vi "RT Main_EVO_V1_chopped_data_V1.vi"(11 "dup Message Queue 2":refnum<queue>) -> ()   [LabVIEW 2017]
uses:
  UI Error Handlers/support/Message Queue/Message Cluster.ctl
  <vilib>/vision/Image Controls.llb/IMAQ Image.ctl
  <vilib>/userdefined/High Color/IMAQdx.ctl
  <vilib>/vision/Avi.llb/IMAQ AVI2 Refnum.ctl
  camera_array_1.ctl
  <vilib>/vision/Avi.llb/IMAQ AVI2 Codec Path.ctl
  Globals/Global - All RT Loop Stop.vi
  Globals/Global - Configuration Options.vi
  <vilib>/vision/driver/NI_Vision_Acquisition_Software.lvlib
  UI Error Handlers/support/Message Queue/Message Queue.lvlib
panel:
  in  "Boolean":bool
  out "Array":T1[](array[typedef])
  out "Webcam":T1(plugin-control)
  out "Codec Names 2":string[](array[string])
  out "concatenated string 4":string
  out "error out":errorcluster
  out "x-y":u32
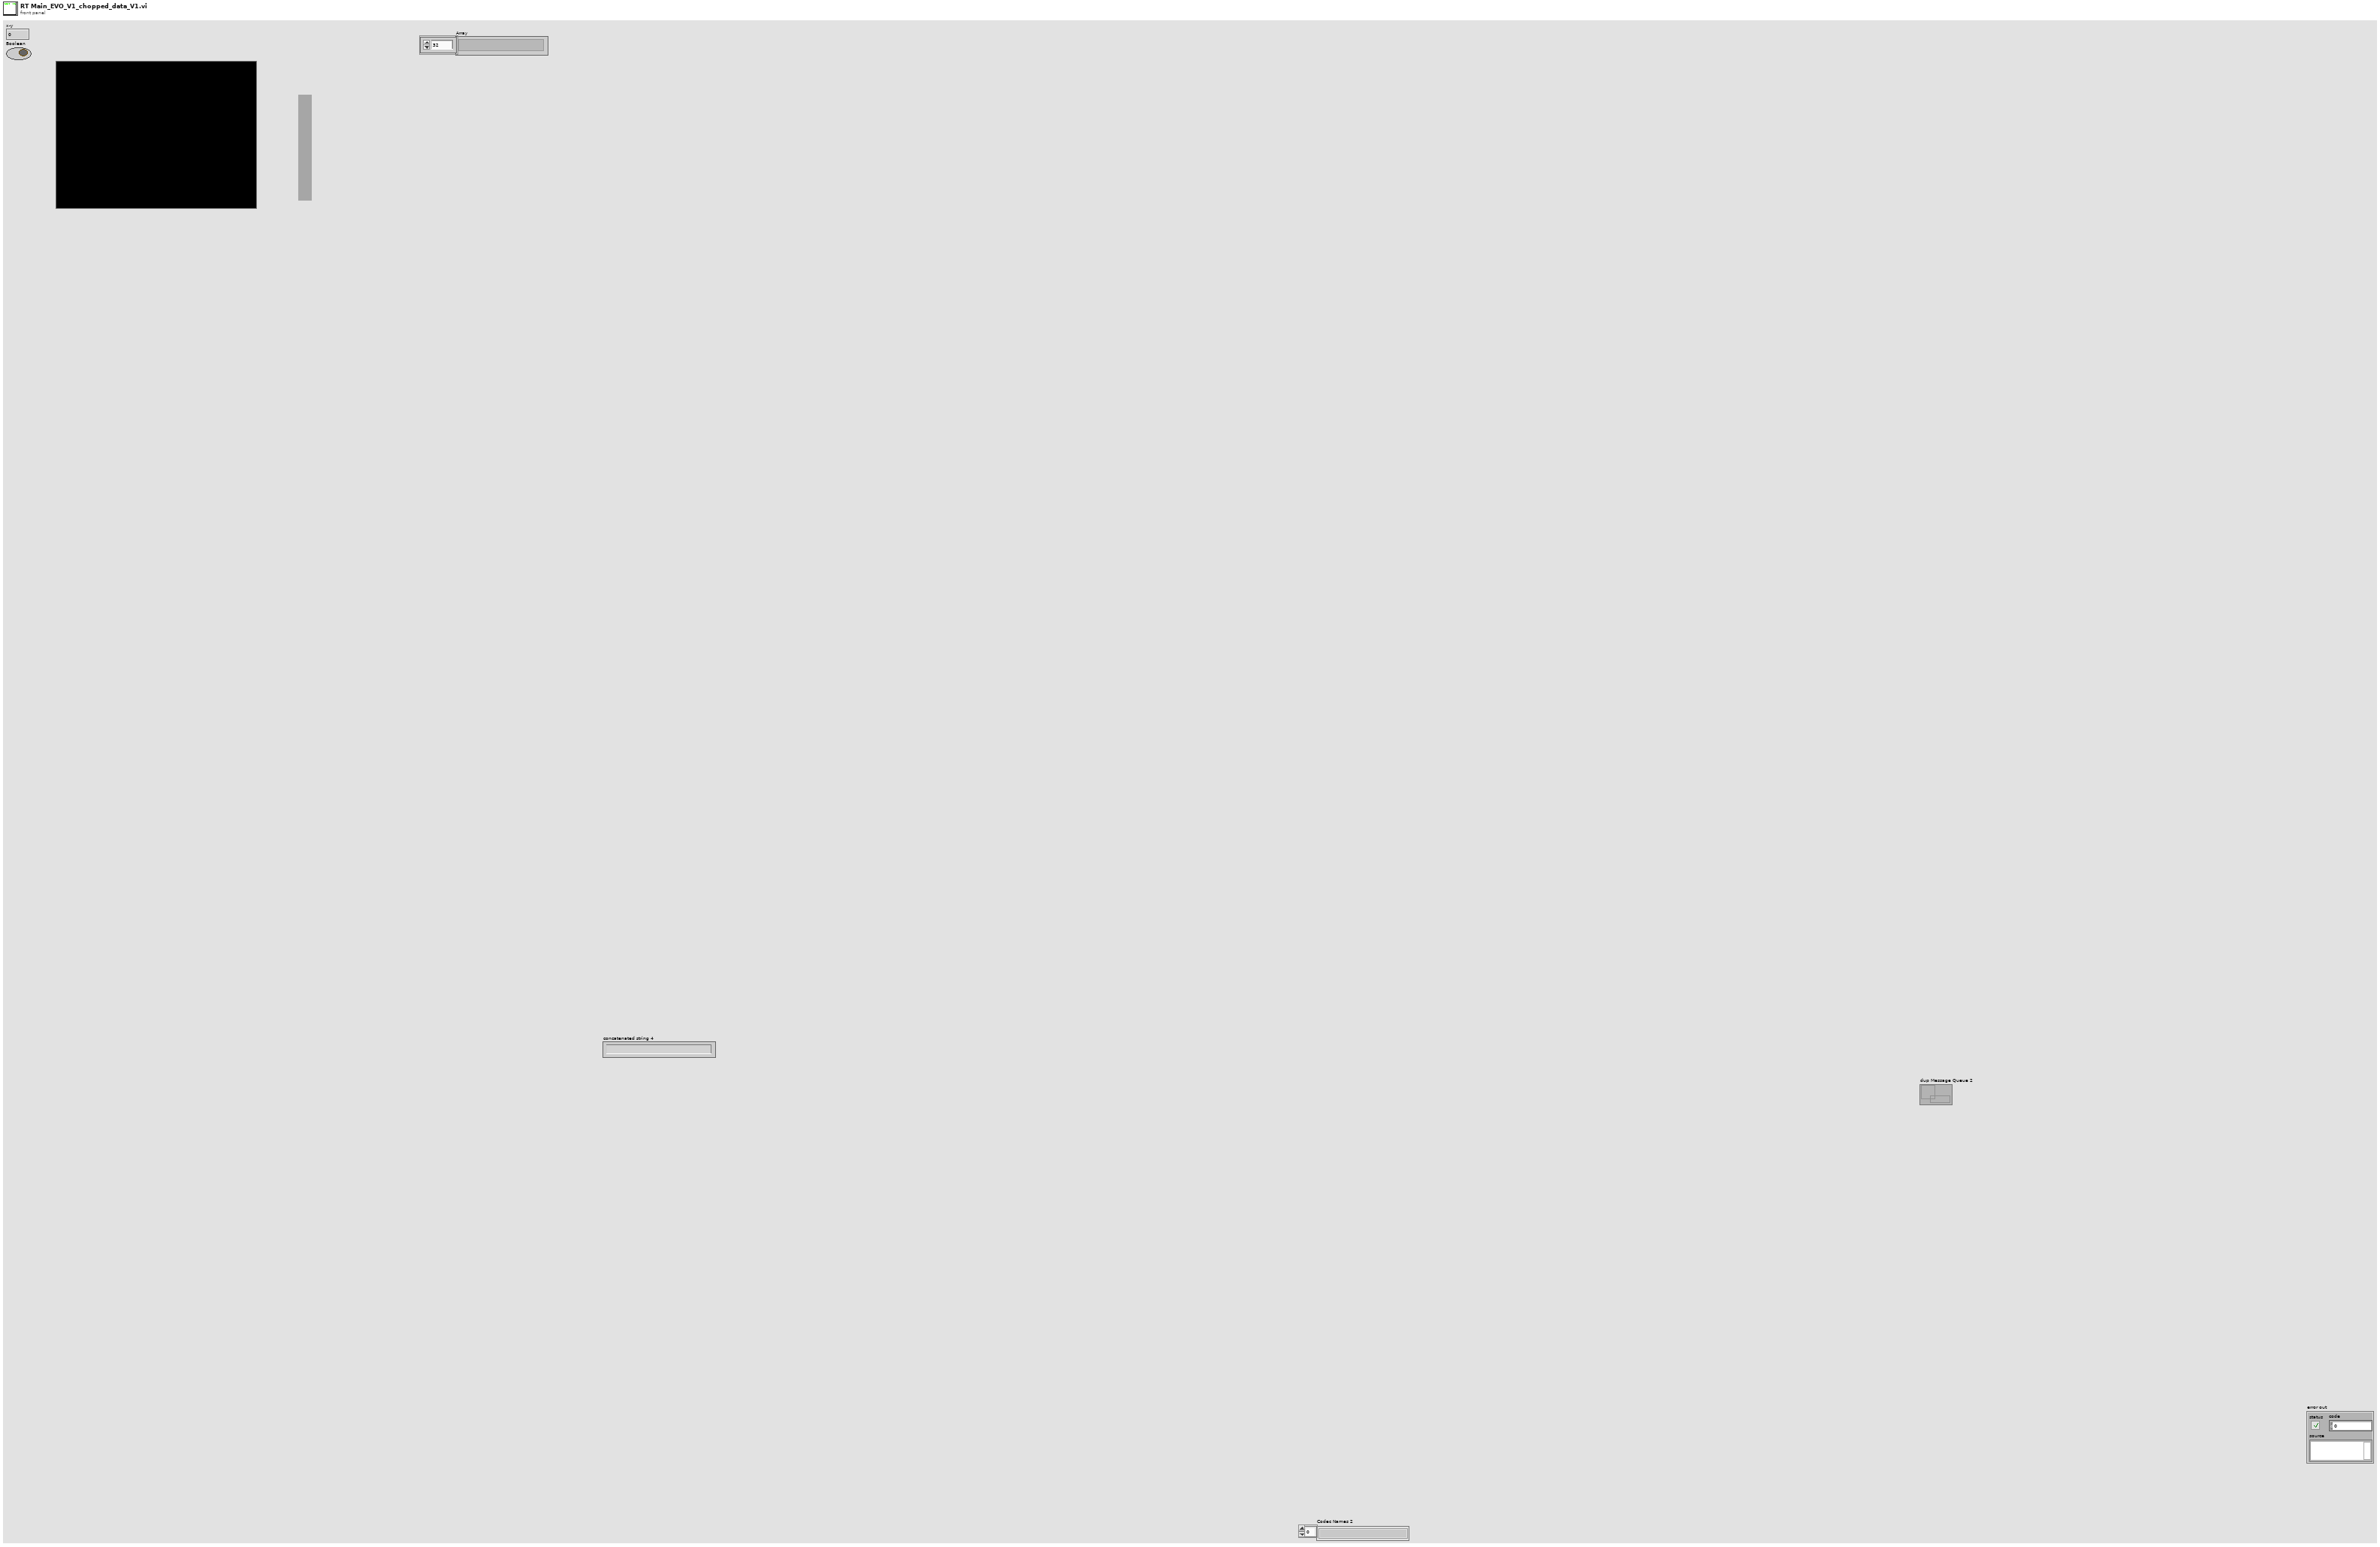
[diagram p1: front panel]
types:
  T1 = typedef "IMAQ Image.ctl" = refnum<image>
  T2 = typedef "camera_array_1.ctl" = T1[]
  T3 = typedef "IMAQ AVI2 Refnum.ctl" = refnum<k20>
  T4 = typedef "IMAQdx.ctl" = refnum<k21>
  T5 = typedef "Image Type" = u32
  T6 = cluster{"Tool data":cluster{"Number of teeth":sgl}, "Cutting data":cluster{"rpm":sgl}, "Limits":cluster{"Magnitude threshold":sgl, "Tolerance":sgl}, "G1 status":cluster{"G1 trigger":bool}}
  T7 = typedef "IMAQ AVI2 Codec Path.ctl" = u32
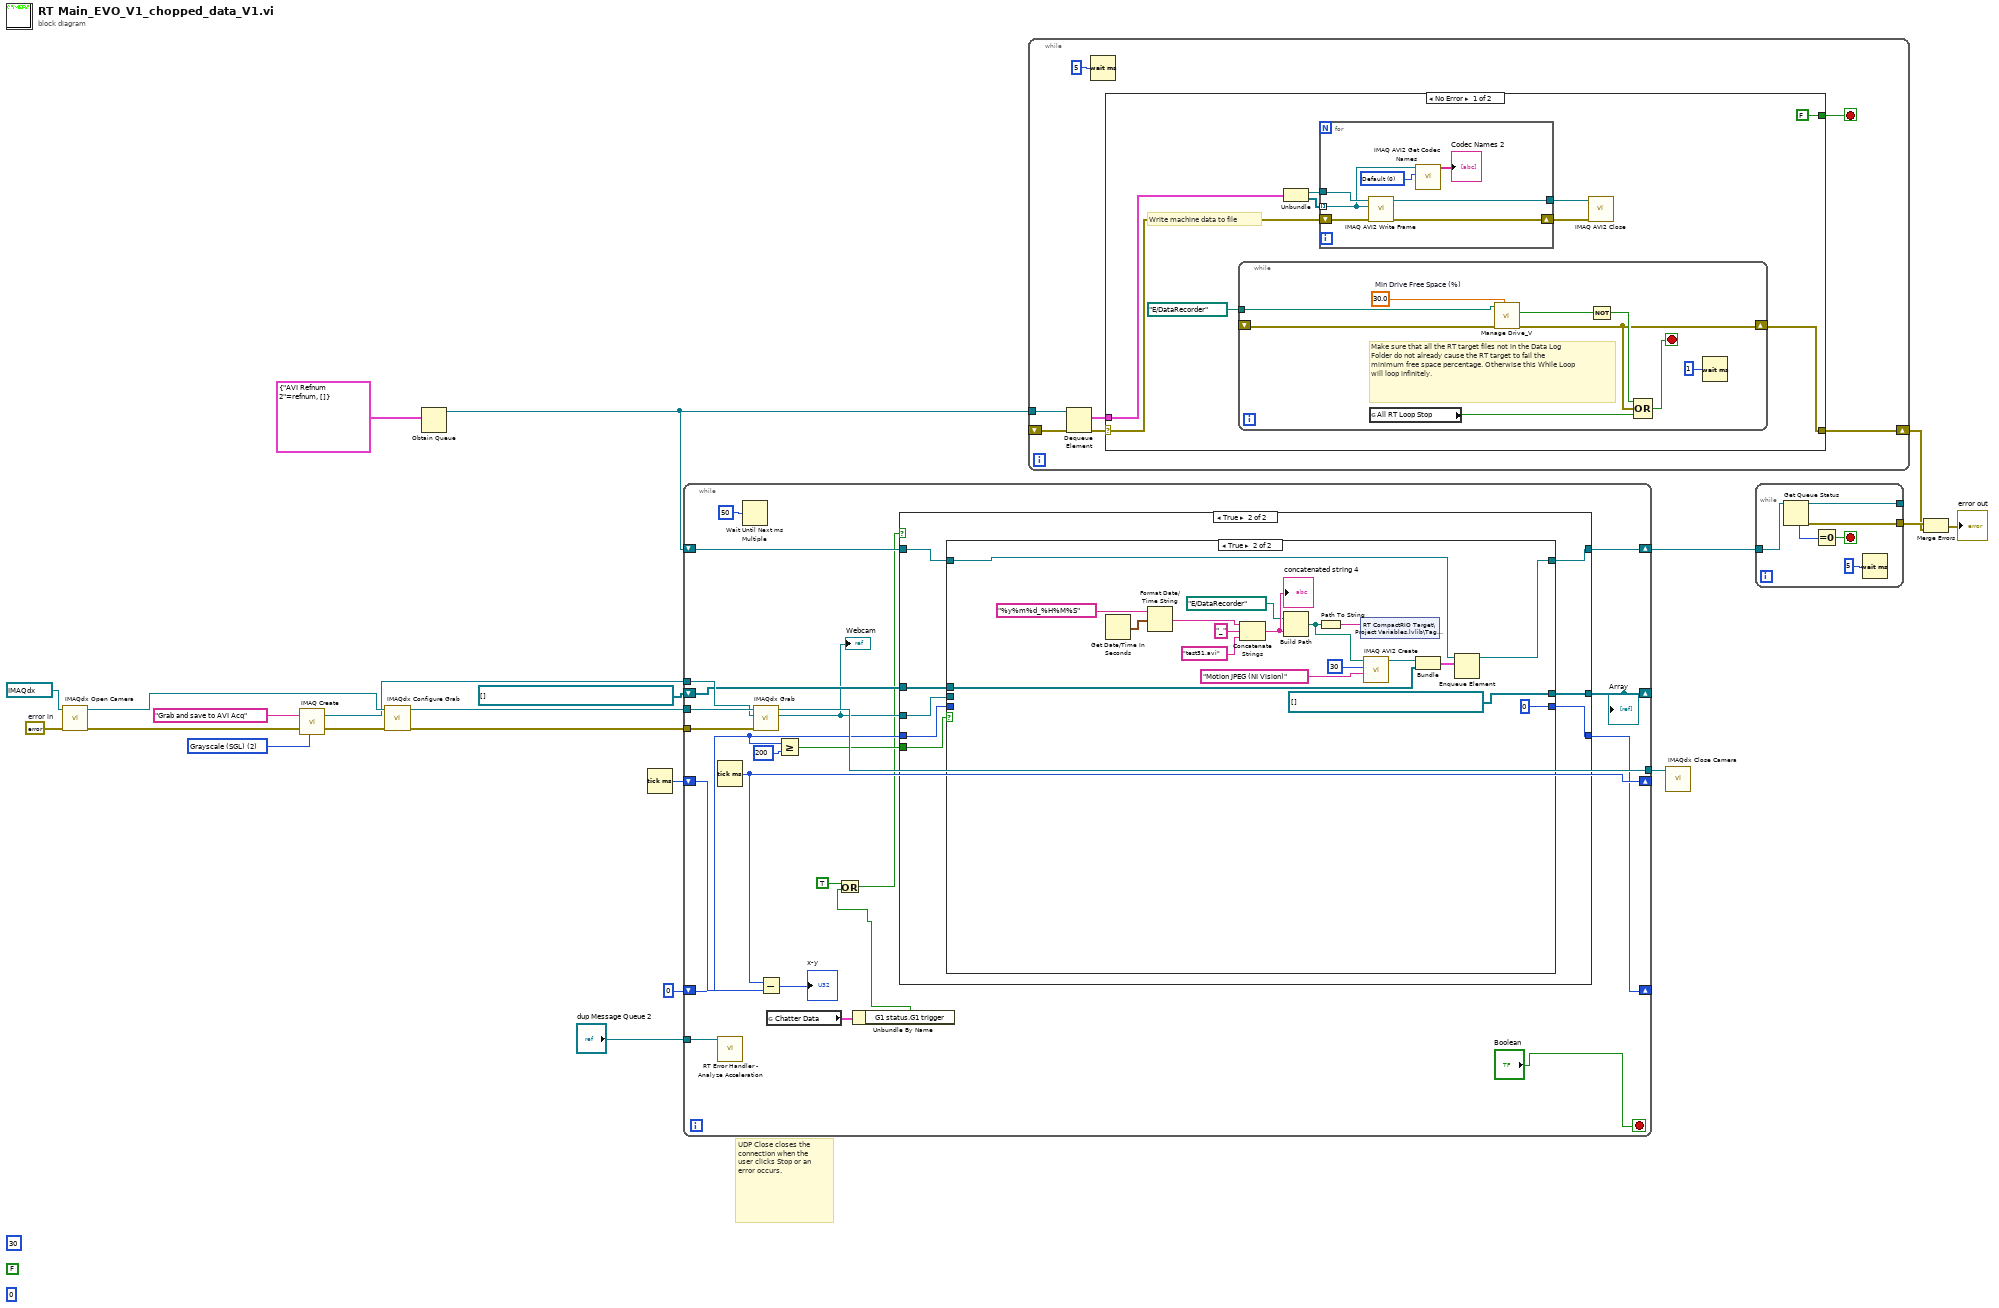
[diagram p0: block diagram]
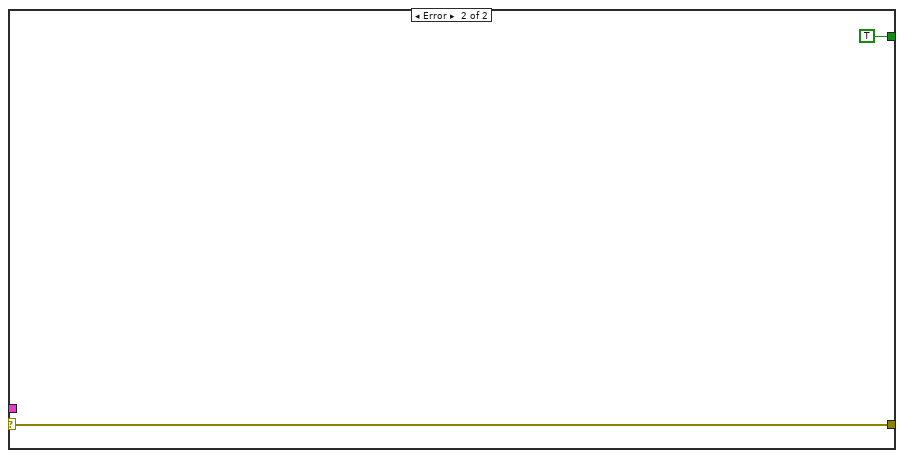
[diagram p2: hidden frame]
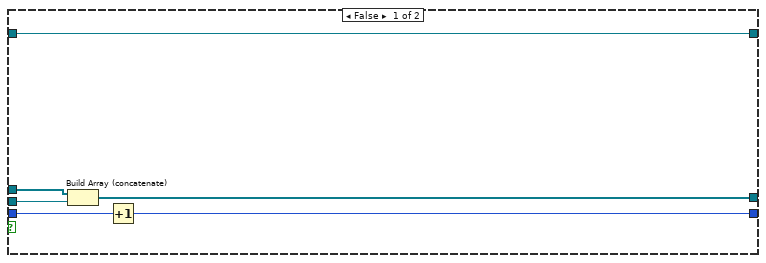
[diagram p4: hidden frame]
diagram:
  w11 = T5 2 items=["Grayscale (U8)", "Grayscale (I16)", "Grayscale (SGL)", "Complex (CSG)", "RGB (U32)", "HSL (U32)", "RGB (U64)", "Grayscale (U16)"] ("Image Type")
  (unwired) u32 30 ("Frames Per Second")
  w12 = errorcluster {"status"=FALSE, "code"=0, "source"=""}  # error in
  (unwired) i16 0 ("A(I16) 11")
  (unwired) FALSE
  # "UDP Close closes the connection when the user clicks Stop or an error occurs."
  n1 = call <vilib>:"IMAQdx Open Camera.vi"("error in"=w12, "Session In"=T4 "cam0") -> ("error out"=w10:errorcluster, "Session Out"=w14:T4)  [unwired: 8 in]
  n2 = call "IMAQ Create"("Image Name"="Grab and save to AVI Acq", "Image Type"=w11, "error in (no error)"=w10) -> ("New Image"=w7:T1, "error out"=w6:errorcluster)  [unwired: 2 in]
  n3 = call <vilib>:"IMAQdx Configure Grab.vi"("error in"=w6, "Session In"=w14) -> ("error out"=w5:errorcluster, "Session Out"=w8:T4)  [unwired: 8 in]
  n4 = Obtain Queue(element data type=cluster{"AVI Refnum 2":T3, T1[]} {"AVI Refnum 2"=refnum, []}) -> (queue out=w19:refnum<queue>)  [unwired: 4 in, 2 out]
  n5 = Tick Count (ms)() -> (millisecond timer value=w15:u32)
  n6 = while {
    shift-right: [w43] -> w21
    shift-left: w19 -> [w44]
    tunnel: "dup Message Queue 2" -> [w42]
    shift-right: [w38] -> _
    shift-left: w15 -> [w39]
    tunnel: w8 -> [w37]
    tunnel: w7 -> [w36]
    tunnel: w5 -> [w35]
    tunnel: [w34] -> w4
    shift-right: [w27] -> _
    shift-left: T2 [] -> [w31]
    shift-right: [w28] -> _
    shift-left: 0 -> [w29]
    stop <- "Boolean" stop-if-true
    n7 = Tick Count (ms)() -> (millisecond timer value=w38:u32)
    n8 = call "RT Error Handler - Analyze Acceleration.vi"("Message Queue"=w42) -> ()  [unwired: 10 in, 1 out]
    n9 = Wait Until Next ms Multiple(millisecond multiple=u32 50) -> ()  [unwired: 1 out]
    n10 = call <vilib>:"IMAQdx Grab.vi"("error in"=w35, "Image In"=w36, "Session In"=w37) -> ("Image Out"=w26:T1, "Session Out"=w34:T4)  [unwired: 5 in, 2 out]
    "Webcam" <- w26
    n11 = Subtract(x=w38, y=w39) -> (x-y=→"x-y":u32)
    n12 = global read "Global - Configuration Options.vi" "Chatter Data"() -> (w41:T6)
    n13 = Greater Or Equal?(x=w29, y=200) -> (x >= y?=w30:bool)
    n14 = Unbundle By Name(w41) -> ("G1 status.G1 trigger"=w25:bool)
    n15 = Or(x=TRUE, y=w25) -> (x .or. y?=w23:bool)
    n16 = case shown="True" w23 {
      tunnel: w44 -> [w47 w48]
      tunnel: [w47 w55] -> w43
      tunnel: w26 -> [_ w54]
      tunnel: w31 -> [w45 w52]
      tunnel: w30 -> [_ w53]
      tunnel: w29 -> [w46 w51]
      tunnel: [w46 w50] -> w28
      tunnel: [w45 w49] -> w27
      frame False {
      }
      frame True {
        n17 = case shown="True" w53 {
          tunnel: [w58 w66] -> w55
          tunnel: w54 -> [w60 _]
          tunnel: w52 -> [w61 w64]
          tunnel: w51 -> [w59 _]
          tunnel: [w57 0] -> w50
          tunnel: [w56 T1[] []] -> w49
          tunnel: w48 -> [w58 w67]
          frame False {
            n18 = Build Array (concatenate)(w61, w60) -> (w56:T2)
            n19 = Increment(x=w59) -> (x+1=w57:i32)
          }
          frame True {
            n20 = Get Date/Time In Seconds() -> (seconds since 1Jan1904=w76:timestamp)
            n21 = Format Date/Time String(time format string (%c)="%y%m%d_%H%M%S", seconds (now)=w76) -> (date/time string=w77:string)  [unwired: 1 out]
            n22 = Concatenate Strings(w77, "_" ("string"), "test51.avi" ("name or relative path")) -> (w78:string)
            "concatenated string 4" <- w78
            n23 = Build Path(base path=path "E:/DataRecorder" ("AVI Path"), name or relative path=w78) -> (appended path=w69:path)
            n24 = Path To String(path=w69) -> (string=w79:string)
            n25 = shared-variable "RT CompactRIO Target\\Project Variables.lvlib\\Tag Video"(w79) -> ()  [unwired: 1 in, 1 out]
            n26 = call "IMAQ AVI2 Create"("Codec"="Motion JPEG (NI Vision)", "Frames Per Second"=u32 30, "AVI Path"=w69) -> ("AVI Refnum"=w65:T3)  [unwired: 7 in, 1 out]
            n27 = Bundle("AVI Refnum"=w65, w64) -> (w63:cluster{"AVI Refnum":T3, T2})  [unwired: 1 in]
            n28 = Enqueue Element(queue=w67, element=w63) -> (queue out=w66:refnum<queue>)  [unwired: 2 in, 2 out]
          }
        }
      }
    }
    "Array" <- w27
  }
  n29 = while {
    tunnel: w19 -> [w86]
    shift-right: [w82] -> w18
    shift-left: _ -> [w85]
    stop <- w83 stop-if-true
    n30 = Dequeue Element(queue=w86, error in (no error)=w85) -> (element=w81:cluster{"AVI Refnum 2":T3, T1[]}, error out=w84:errorcluster)  [unwired: 1 in, 2 out]
    n31 = Wait (ms)(milliseconds to wait=u32 5) -> ()  [unwired: 1 out]
    n32 = case shown="No Error" w84 {
      selector: w84 -> [w94 w112]
      tunnel: [FALSE TRUE] -> w83
      tunnel: [w90 w112] -> w82
      tunnel: w81 -> [w89 _]
      frame No Error {
        # "Write machine data to file"
        n33 = while {
          shift-right: [w106] -> w90
          shift-left: _ -> [w107]
          tunnel: path "E:/DataRecorder" ("AVI Path") -> [w104]
          stop <- w111 stop-if-true
          w105 = 30.0  # Min Drive Free Space (%)
          # "Make sure that all the RT target files not in the Data Log Folder do not already cause the RT target to fail the minimum free space percentage. Otherwise this While Loop will loop infinitely."
          n34 = global read "Global - All RT Loop Stop.vi" "All RT Loop Stop"() -> (w108:bool)
          n35 = call "Manage Drive_V.vi"("Min Drive Free Space (%)"=w105, "error in"=w107, "Data Folder"=w104) -> ("error out"=w106:errorcluster, "Drive Space Below Limit"=w103:bool)  [unwired: 6 in, 1 out]
          n36 = Not(x=w103) -> (.not. x?=w110:bool)
          n37 = Compound Arithmetic op=OR(w110, w106, w108) -> (w111:bool)
          n38 = Wait (ms)(milliseconds to wait=u32 1) -> ()  [unwired: 1 out]
        }
        n39 = Unbundle(w89) -> ("AVI Refnum 2"=w88:T3, w87:T1[])
        n40 = for {
          shift-right: [w100] -> w92
          shift-left: w94 -> [w102]
          tunnel: w88 -> [w99]
          tunnel: [w101] -> w93
          tunnel: w87 -> [w96] mode=indexing
          w98 = T7 0 items=["Default", "System", "Built in Vision"] ("Codec Source")
          n41 = call "IMAQ AVI2 Write Frame"("error in (no error)"=w102, "Image"=w96, "AVI Refnum"=w99) -> ("error out"=w100:errorcluster, "AVI Refnum (duplicate)"=w101:T3)  [unwired: 6 in, 1 out]
          n42 = call "IMAQ AVI2 Get Codec Names"("Codec Source"=w98, "Image"=w96) -> ("Codec Names"=→"Codec Names 2":string[])  [unwired: 8 in, 1 out]
        }
        n43 = call "IMAQ AVI2 Close"("error in (no error)"=w92, "AVI Refnum"=w93) -> ()  [unwired: 9 in, 1 out]
      }
      frame Error {
      }
    }
  }
  n44 = call <vilib>:"IMAQdx Close Camera.vi"("Session In"=w4) -> ()  [unwired: 10 in, 1 out]
  n45 = while {
    tunnel: [w118] -> w20
    tunnel: [w116] -> _
    tunnel: w21 -> [w114]
    stop <- w117 stop-if-true
    n46 = Get Queue Status(queue=w114) -> (queue out=w116:refnum<queue>, error out=w118:errorcluster, # elements in queue=w115:i32)  [unwired: 2 in, 5 out]
    n47 = Equal To 0?(x=w115) -> (x = 0?=w117:bool)
    n48 = Wait (ms)(milliseconds to wait=u32 5) -> ()  [unwired: 1 out]
  }
  n49 = Merge Errors(w20, w18) -> (→"error out":errorcluster)
